vi "Parker_Gen2Sensor_v2.3.vi"(0 "Com Port":refnum<visa-resource-name>="COM5") -> (9 "Raw Serial Data":string="\r\n")   [LabVIEW 2015]
doc: "The Basic Serial Read and Write example performs a Serial Port Read, a Serial Port Write, or a combination of these actions. The user selects the actions (read or write) on the front panel. If both are selected, the VI will write the data first, read data, and then close the VISA session that is opened to the port. This VI will wait until the specified number of bytes is received at the port or until a termination character is read.\n\nINSTRUCTIONS:\n1) Select the serial resource and configuration parameters (baud rate, data bits, parity, stop bits, flow control).\n2) Select the operations to be performed. \n3) Connect the serial port to your device. If no device is available, perform a loopback test by doing one of the following. Short pins 2 and 3 on a RS-232 cable or short pin 4 to pin 8 and pin 5 to pin 9 on a RS-485/422 cable. \n4) Run the VI to see the data read. (The \"read string\" will match the \"string to write\" if a loopback test was performed.)\n\nNote: The parameters set for the serial port must match the parameters of the connected instrument or device. In this example, the bytes to read parameter specifies the number of bytes that the serial port reads. If there were more bytes at the port than the number specified in bytes to read, those bytes would not be read. Also, if you specify to read more bytes than the number of bytes actually read, you might receive a timeout error message.\n\nOn the block diagram, the Configure Serial Port VI sets the configuration parameters. The front panel displays the controls used to configure the basic parameters, such as baud rate, data bits, and parity. Constants configure the other parameters the user probably does not need set. After the VISA Configure Serial Port VI opens the VISA session and configures the port, the VI passes the VISA resource name to other VIs that perform operations on that VISA resource. The VISA Write function sends a command to the serial device and the VISA Read function returns data based on the command. The VISA Close function then closes the reference to the serial device. It is important to close the reference; otherwise communication through with that port through protocols other than VISA might not be possible."
uses:
  <vilib>/Utility/error.llb/DialogType.ctl
  <vilib>/Instr/_visa.llb/VISA Configure Serial Port (Instr).vi
  <vilib>/Utility/file.llb/Write Delimited Spreadsheet (DBL).vi
panel:
  in  "Reset":bool
  in  "100%":bool
  in  "Zero":bool
  in  "Full Stretch Value":dbl=100.0
  in  "Zero Value":dbl
  in  "Exit Program":bool
  in  "Stop Program":bool
  in  "Start Program":bool
  out "Temperature":dbl=299.0
  out "Sensor Value":dbl=2.0
  out "Adjusted Sensor Output":dbl(graph)=1.94
  out "Sensor Ouput":dbl(graph)=1.94
  # "Operating Insructions:\n1) Select appropriate COM port\n2) Push \"Start Program\"\n3) Push \"Stop Program\" when finished. \n      User will be prompted to save data or not."
  # "Main\nControls"
  # "Calibration"
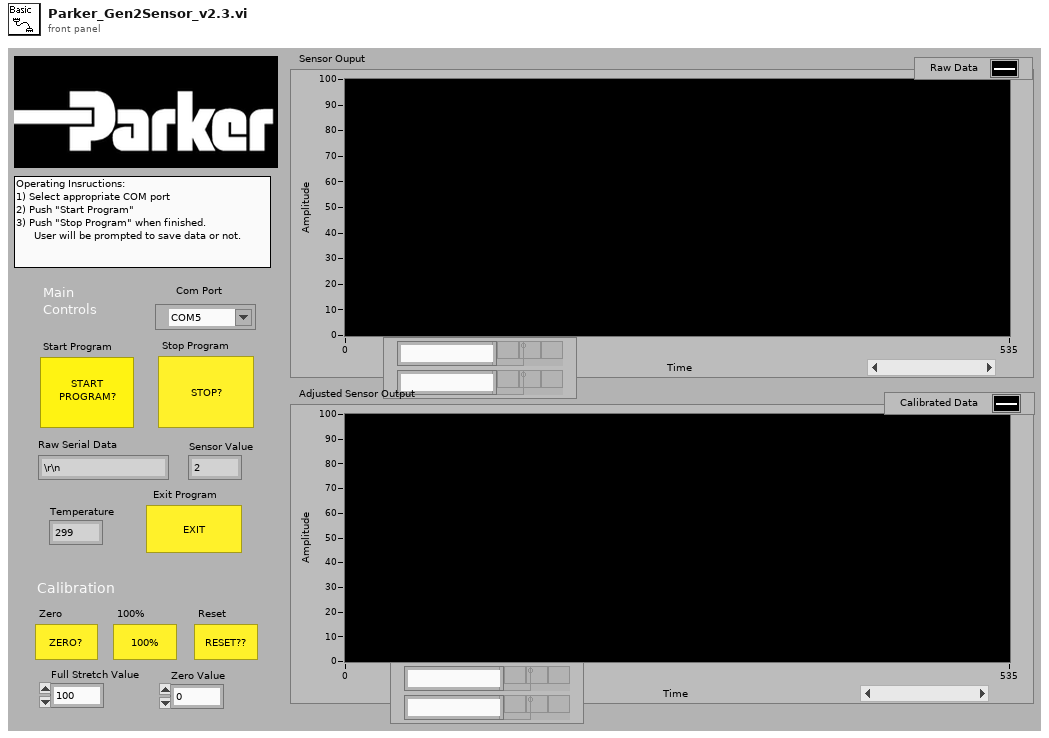
[diagram p1: front panel]
types:
  T1 = enum8{"Enabled", "Disabled", "Disabled and Grayed Out"}
  T2 = typedef "DialogType.ctl" = u16
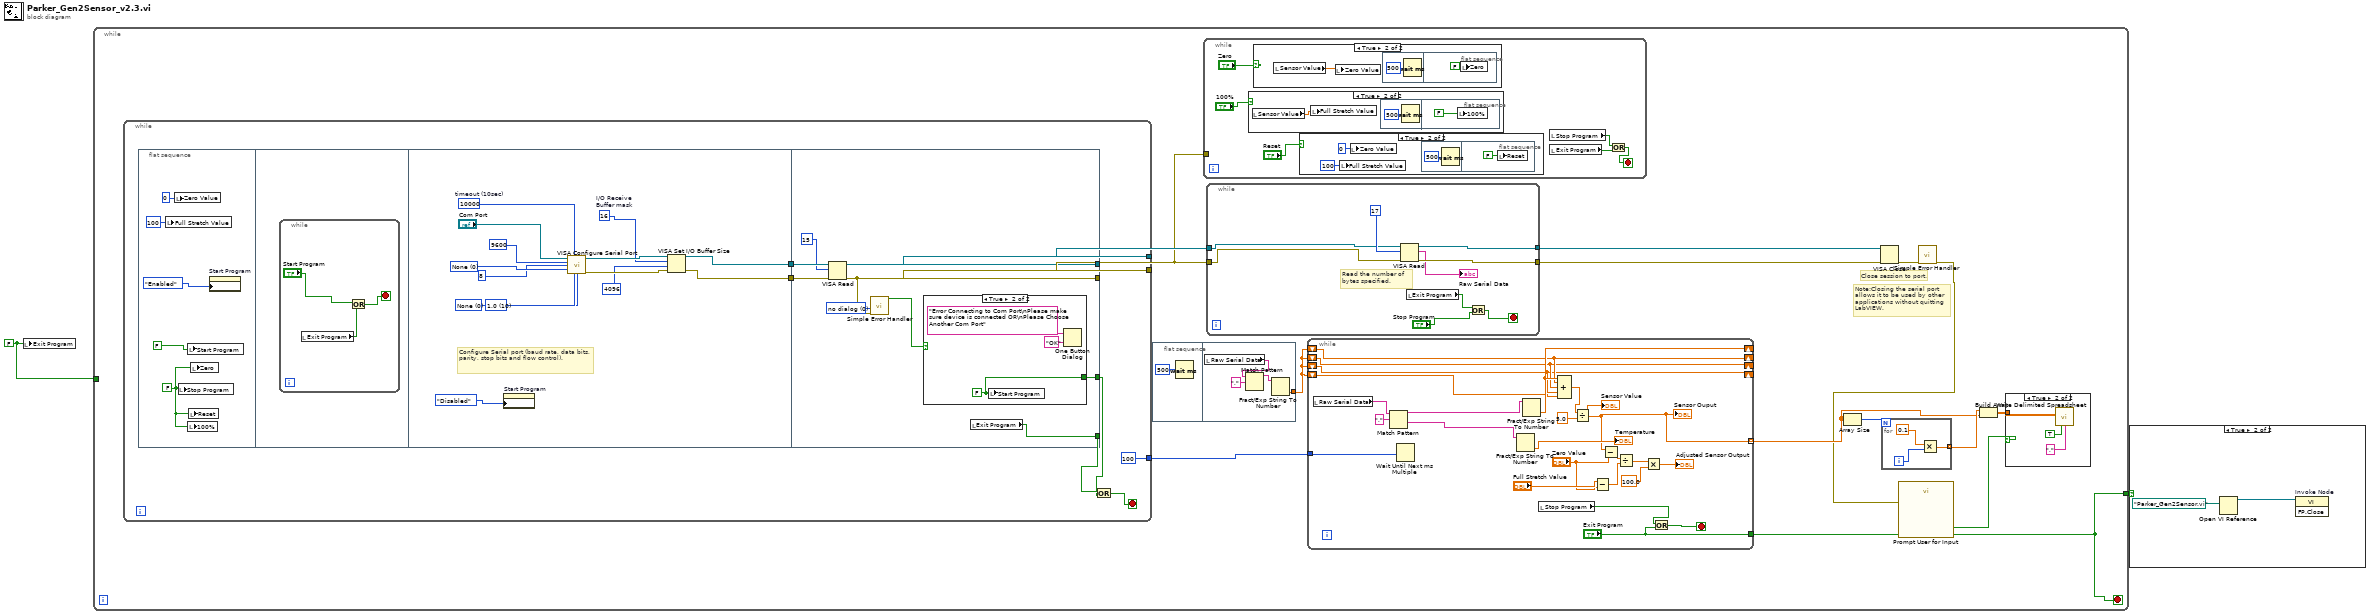
[diagram p0: block diagram]
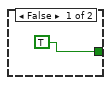
[diagram p7: hidden frame]
diagram:
  w2 = FALSE ("END PROGRAM")
  n1 = local write "Exit Program"(w2) -> ()
  n2 = while {
    tunnel: w2 -> [_]
    tunnel: [w5] -> w1
    stop <- w5 stop-if-true
    # "Note:Closing the serial port allows it to be used by other applications without quitting LabVIEW."
    # "Close session to port."
    n3 = while {
      tunnel: [w51] -> w4
      tunnel: [w50] -> w13
      tunnel: [u32 100 ("millisecond multiple")] -> w12
      stop <- w45 stop-if-true
      n4 = flat-sequence {
        tunnel: [w64] -> w49
        tunnel: [w63] -> w48
        tunnel: [w78] -> w50
        tunnel: [w79] -> w51
        tunnel: w49 -> [w80]
        tunnel: w48 -> [w81]
        tunnel: [w76] -> w44
        tunnel: [w74] -> w46
        frame #0 {
          w54 = FALSE
          n5 = local write "Full Stretch Value"(100 ("Full Stretch Value")) -> ()
          n6 = local write "Zero Value"(0 ("Zero Value")) -> ()
          n7 = local write "Stop Program"(w54) -> ()
          n8 = local write "Start Program"(FALSE) -> ()
          n9 = local write "100%"(w54) -> ()
          n10 = local write "Reset"(w54) -> ()
          n11 = local write "Zero"(w54) -> ()
          n12 = property on="Start Program" class="Bool (strict)"("DisabledEnum"=T1."Enabled" ("Disabled")) -> ()  [unwired: 2 in, 2 out]
        }
        frame #1 {
          n13 = while {
            stop <- w57 stop-if-true
            n14 = local read "Exit Program"() -> (w58:bool)
            n15 = Or(x="Start Program", y=w58) -> (x .or. y?=w57:bool)
          }
        }
        frame #2 {
          w68 = u16 0 items=["None"=0, "XON/XOFF"=1, "RTS/CTS"=2, "DTR/DSR"=4] ("flow control")
          w69 = u16 10 items=["1.0"=10, "1.5"=15, "2.0"=20] ("stop bits")
          w71 = u16 0 items=["None", "Odd", "Even", "Mark", "Space"] ("parity")
          w62 = u16 16  # I/O Receive Buffer mask
          w70 = u32 10000  # timeout (10sec)
          # "Configure Serial port (baud rate, data bits, parity, stop bits and flow control)."
          n16 = property on="Start Program" class="Bool (strict)"("DisabledEnum"=T1."Disabled" ("Disabled")) -> ()  [unwired: 2 in, 2 out]
          n17 = call-poly "VISA Configure Serial Port"("VISA resource name"="Com Port", "timeout (10sec)"=w70, "baud rate (9600)"=u32 9600 ("baud rate"), "data bits (8)"=u16 8 ("data bits"), "parity (0:none)"=w71, "stop bits (10: 1 bit)"=w69, "flow control (0:none)"=w68) -> ("VISA resource name out"=w66:refnum<visa-resource-name>, "error out"=w65:errorcluster)  [unwired: 2 in, 5 out]
          n18 = VISA Set I/O Buffer Size(VISA resource name=w66, mask (16)=w62, size (4096)=u32 4096 ("Input\nbuffer size"), error in (no error)=w65) -> (VISA resource name out=w63:refnum<visa-resource-name>, error out=w64:errorcluster)
        }
        frame #3 {
          w82 = T2 0 items=["no dialog", "OK message", "continue or stop message", "OK message + warnings", "continue/stop + warnings"] ("type of dialog (OK msg:1)")
          n19 = VISA Read(VISA resource name=w81, byte count=u32 15 ("bytes read"), error in (no error)=w80) -> (VISA resource name out=w78:refnum<visa-resource-name>, error out=w79:errorcluster)  [unwired: 2 out]
          n20 = call <vilib>:"Simple Error Handler.vi"("type of dialog (OK msg:1)"=w82, "error in (no error)"=w79) -> ("error?"=w77:bool)  [unwired: 7 out]
          n21 = case shown="True" w77 {
            tunnel: [TRUE w84] -> w76
            frame False {
            }
            frame True {
              w84 = FALSE ("Start Program")
              n22 = local write "Start Program"(w84) -> ()
              n23 = One Button Dialog(message="Error Connecting to Com Port\nPlease make sure device is connected OR\nPlease Choose Another Com Port", button name ("OK")="OK") -> ()  [unwired: 1 out]
            }
          }
          n24 = local read "Exit Program"() -> (w74:bool)
        }
      }
      n25 = Or(x=w46, y=w44) -> (x .or. y?=w45:bool)
    }
    n26 = flat-sequence {
      tunnel: [w19] -> w3
      frame #0 {
        n27 = Wait (ms)(milliseconds to wait=u32 500) -> ()  [unwired: 1 out]
      }
      frame #1 {
        n28 = local read "Raw Serial Data"() -> (w18:string)
        n29 = Match Pattern(string=w18, regular expression=",") -> (before substring=w20:string)  [unwired: 1 in, 3 out]
        n30 = Fract/Exp String To Number(string=w20) -> (number=w19:dbl)  [unwired: 3 in, 1 out]
      }
    }
    n31 = while {
      tunnel: w4 -> [_]
      stop <- w27 stop-if-true
      n32 = case shown="True" "100%" {
        frame False {
        }
        frame True {
          n33 = local read "Sensor Value"() -> (w32:dbl)
          n34 = local write "Full Stretch Value"(w32) -> ()
          n35 = flat-sequence {
            frame #0 {
              n36 = Wait (ms)(milliseconds to wait=u32 500) -> ()  [unwired: 1 out]
            }
            frame #1 {
              n37 = local write "100%"(FALSE ("Full Stretch")) -> ()
            }
          }
        }
      }
      n38 = case shown="True" "Zero" {
        frame False {
        }
        frame True {
          n39 = local read "Sensor Value"() -> (w35:dbl)
          n40 = local write "Zero Value"(w35) -> ()
          n41 = flat-sequence {
            frame #0 {
              n42 = Wait (ms)(milliseconds to wait=u32 500) -> ()  [unwired: 1 out]
            }
            frame #1 {
              n43 = local write "Zero"(FALSE) -> ()
            }
          }
        }
      }
      n44 = case shown="True" "Reset" {
        frame False {
        }
        frame True {
          n45 = local write "Full Stretch Value"(100 ("Full Stretch Value")) -> ()
          n46 = local write "Zero Value"(0 ("Zero Value")) -> ()
          n47 = flat-sequence {
            frame #0 {
              n48 = Wait (ms)(milliseconds to wait=u32 500) -> ()  [unwired: 1 out]
            }
            frame #1 {
              n49 = local write "Reset"(FALSE ("Reset")) -> ()
            }
          }
        }
      }
      n50 = local read "Stop Program"() -> (w26:bool)
      n51 = local read "Exit Program"() -> (w25:bool)
      n52 = Or(x=w26, y=w25) -> (x .or. y?=w27:bool)
    }
    n53 = while {
      tunnel: w4 -> [w114]
      tunnel: w13 -> [w115]
      tunnel: [w119] -> w16
      tunnel: [w118] -> w15
      stop <- w112 stop-if-true
      # "Read the number of bytes specified."
      n54 = VISA Read(VISA resource name=w115, byte count=u32 17 ("bytes read"), error in (no error)=w114) -> (VISA resource name out=w118:refnum<visa-resource-name>, read buffer=→"Raw Serial Data":string, error out=w119:errorcluster)  [unwired: 1 out]
      n55 = local read "Exit Program"() -> (w111:bool)
      n56 = Or(x=w111, y="Stop Program") -> (x .or. y?=w112:bool)
    }
    n57 = while {
      tunnel: w12 -> [w107]
      tunnel: [w88] -> w9 mode=indexing
      tunnel: ["Exit Program"] -> w5
      shift-right: [w94] -> _
      shift-left: w3 -> [w93]
      shift-right: [w93] -> _
      shift-left: w3 -> [w92]
      shift-right: [w92] -> _
      shift-left: w3 -> [w91]
      shift-right: [w91] -> _
      shift-left: w3 -> [w90]
      stop <- w105 stop-if-true
      n58 = local read "Raw Serial Data"() -> (w108:string)
      n59 = Match Pattern(string=w108, regular expression=",") -> (before substring=w109:string, after substring=w96:string)  [unwired: 1 in, 2 out]
      n60 = Wait Until Next ms Multiple(millisecond multiple=w107) -> ()  [unwired: 1 out]
      n61 = Fract/Exp String To Number(string=w96) -> (number=→"Temperature":dbl)  [unwired: 3 in, 1 out]
      n62 = Fract/Exp String To Number(string=w109) -> (number=w94:dbl)  [unwired: 3 in, 1 out]
      n63 = local read "Stop Program"() -> (w106:bool)
      n64 = Compound Arithmetic op=ADD(w94, w93, w92, w91, w90) -> (w89:dbl)
      n65 = Divide(x=w89, y=5.0) -> (x/y=w88:dbl)
      "Sensor Value" <- w88
      "Sensor Ouput" <- w88
      n66 = Subtract(x="Full Stretch Value", y="Zero Value") -> (x-y=w97:dbl)
      n67 = Subtract(x=w88, y="Zero Value") -> (x-y=w100:dbl)
      n68 = Divide(x=w100, y=w97) -> (x/y=w101:dbl)
      n69 = Multiply(x=w101, y=100.0) -> (x*y=→"Adjusted Sensor Output":dbl)
      n70 = Or(x=w106, y="Exit Program") -> (x .or. y?=w105:bool)
    }
    n71 = Array Size(array=w9) -> (size(s)=w11:i32)
    n72 = VISA Close(VISA resource name=w15, error in (no error)=w16) -> (error out=w14:errorcluster)
    n73 = for {
      N: w11 -> [_]
      tunnel: [w41] -> w10 mode=indexing
      i -> [w43]
      n74 = Multiply(x=0.1, y=w43) -> (x*y=w41:dbl)
    }
    n75 = call <vilib>:"Simple Error Handler.vi"("error in (no error)"=w14) -> ("error out"=w6:errorcluster)  [unwired: 1 in, 7 out]
    n76 = call "Prompt User for Input"("error in (no error)"=w6) -> ("YES"=w7:bool)  [unwired: 17 in, 1 out]
    n77 = Build Array(w10, w9) -> (w8:dbl[][])
    n78 = case shown="True" w7 {
      tunnel: w8 -> [_ w40]
      frame False {
      }
      frame True {
        n79 = call-poly <vilib>:"Write Delimited Spreadsheet.vi"("2D data"=w40, "transpose? (F)"=TRUE, "delimiter (\\t)"="," ("delimiter (\\t)")) -> ()  [unwired: 11 in, 2 out]
      }
    }
  }
  n80 = case shown="True" w1 {
    frame False {
    }
    frame True {
      n81 = Open VI Reference(vi path=path "Parker_Gen2Sensor.vi") -> (vi reference=w120:refnum<vi>)  [unwired: 5 in, 1 out]
      n82 = invoke on="Invoke Node" class="VI" method="FP.Close"(reference=w120) -> ()  [unwired: 2 in, 3 out]
    }
  }
